vi "dfd_Validate Filter Bank.vi"(8 "error in (no error)":errorcluster, 11 "filter banks in":T1 {"mFBank_SynthesisFilters"."mMRate_SumWl" min=1 max=32 step=1; "mFBank_SynthesisFilters"."mMRate_InputIwl" min=1 max=32 step=1; "mFBank_SynthesisFilters"."mMRate_GainWl" min=1 max=32 step=1; "mFBank_SynthesisFilters"."mMRate_OutputWl" min=1 max=32 step=1; "mFBank_SynthesisFilters"."mMRate_InputWl" min=1 max=32 step=1; "mFBank_SynthesisFilters"."mMRate_CoefWl" min=1 max=32 step=1; "mFBank_SynthesisFilters"."mMRate_Mode" items=["Default"=-1, "No Rate Change"=0, "Interpolation"=1, "Decimation"=2, "Interpolated"=3, "Rational"=4]; "mFBank_AnalysisFilters"."mMRate_SumWl" min=1 max=32 step=1; "mFBank_AnalysisFilters"."mMRate_InputIwl" min=1 max=32 step=1; "mFBank_AnalysisFilters"."mMRate_GainWl" min=1 max=32 step=1; "mFBank_AnalysisFilters"."mMRate_OutputWl" min=1 max=32 step=1; "mFBank_AnalysisFilters"."mMRate_InputWl" min=1 max=32 step=1; "mFBank_AnalysisFilters"."mMRate_CoefWl" min=1 max=32 step=1; "mFBank_AnalysisFilters"."mMRate_Mode" items=["Default"=-1, "No Rate Change"=0, "Interpolation"=1, "Decimation"=2, "Interpolated"=3, "Rational"=4]; "mFBank_Type" items=["Uniform", "Non-Uniform"]}) -> (0 "error out":errorcluster, 2 "is Valid?":bool, 3 "filter bank out":T1 {"mFBank_SynthesisFilters"."mMRate_SumWl" min=1 max=32 step=1; "mFBank_SynthesisFilters"."mMRate_InputIwl" min=1 max=32 step=1; "mFBank_SynthesisFilters"."mMRate_GainWl" min=1 max=32 step=1; "mFBank_SynthesisFilters"."mMRate_OutputWl" min=1 max=32 step=1; "mFBank_SynthesisFilters"."mMRate_InputWl" min=1 max=32 step=1; "mFBank_SynthesisFilters"."mMRate_CoefWl" min=1 max=32 step=1; "mFBank_SynthesisFilters"."mMRate_Mode" items=["Default"=-1, "No Rate Change"=0, "Interpolation"=1, "Decimation"=2, "Interpolated"=3, "Rational"=4]; "mFBank_AnalysisFilters"."mMRate_SumWl" min=1 max=32 step=1; "mFBank_AnalysisFilters"."mMRate_InputIwl" min=1 max=32 step=1; "mFBank_AnalysisFilters"."mMRate_GainWl" min=1 max=32 step=1; "mFBank_AnalysisFilters"."mMRate_OutputWl" min=1 max=32 step=1; "mFBank_AnalysisFilters"."mMRate_InputWl" min=1 max=32 step=1; "mFBank_AnalysisFilters"."mMRate_CoefWl" min=1 max=32 step=1; "mFBank_AnalysisFilters"."mMRate_Mode" items=["Default"=-1, "No Rate Change"=0, "Interpolation"=1, "Decimation"=2, "Interpolated"=3, "Rational"=4]; "mFBank_Type" items=["Uniform", "Non-Uniform"]})   [LabVIEW 2017, in "NI_DigFilter_FilterBank.lvlib"]
uses:
  <vilib>/addons/Digital Filter Design/NI_DigFilter_FilterBank.lvlib
  <vilib>/addons/Digital Filter Design/FilterBank.llb/Object/DFD Filter Bank Obj.ctl
  <vilib>/addons/Digital Filter Design/_Objects.llb/DFD Multirate Filter Obj.ctl
  <vilib>/addons/Digital Filter Design/_Objects.llb/DFD Multirate Mode.ctl
  <vilib>/addons/Digital Filter Design/_Objects.llb/DFD Coef Norm Type.ctl
  <vilib>/addons/Digital Filter Design/_Objects.llb/DFD Round-off Mode.ctl
  <vilib>/addons/Digital Filter Design/_Objects.llb/DFD FXP MRate Multiply Mode.ctl
  <vilib>/addons/Digital Filter Design/FilterBank.llb/Object/DFD Filter Bank Processing Method.ctl
  <vilib>/addons/Digital Filter Design/FilterBank.llb/Object/DFD Filter Bank Type.ctl
  <vilib>/addons/Digital Filter Design/_Misc.llb/dfd_Error Handlers (Single).vi
  <vilib>/addons/Digital Filter Design/NI_DigFilterLicensed.lvlib
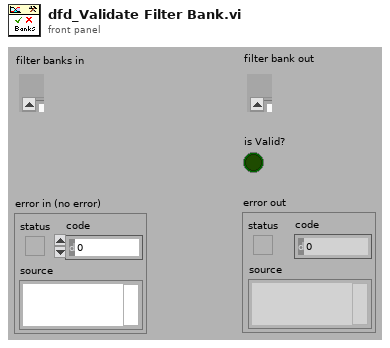
[diagram p1: front panel]
types:
  T1 = typedef "NI_DigFilter_FilterBank.lvlib/DFD Filter Bank Obj.ctl" = cluster{"mFBank_AnalysisFilters":T2[], "mFBank_SynthesisFilters":T2[], "mFBank_#Bands":i32, "mFBank_ProcMethod":T7, "mFBank_Coeffs":dbl[], "mFBank_Gain":dbl, "mFBank_Delay":i32, "mFBank_Type":T8}
  T2 = typedef "NI_DigFilterLicensed.lvlib/DFD Multirate Filter Obj.ctl" = cluster{"mMRate_Structure":enum16{"CIC", "FIR", "IIR", "Lattice"}, "mMRate_Mode":T3, "mMRate_Factor":i32, "mMRate_FIRParams":cluster{"mMRate_FIR_H":dbl[], "mMRate_FIR_IsNyquist?":bool, "mMRate_FIR_IsSymmetric?":bool}, "mMRate_CICParams":cluster{"mMRate_CIC_#Stage":i32, "mMRate_CIC_Lag":i32, "mMRate_CIC_Type":enum16{"Lowpass", "Highpass"}}, "mMRate_Order":i32, "mMRate_Version":string, "mMRate_Comments":string, "mMRate_RationalFactor":cluster{"mMRate_L":i32, "mMRate_M":i32}, "mMRate_Fs":dbl, "mMRate_Quantized?":bool, "mMRate_QFilterGain":dbl, "mMRate_CoefWl":i16, "mMRate_Scaling":cluster{"mMRate_ScaleByPowerOf2?":bool, "mMRate_ScaleType":T4}, "mMRate_InputWl":i16, "mMRate_OutputWl":i16, "mMRate_OutputMode":T5, "mMRate_MultMode":T6, "mMRate_BitPruning":bool, "mMRate_GainWl":i16, "mMRate_OutputFwl":i16, "mMRate_SumIwl":i16, "mMRate_InputIwl ":i16, "mMRate_SumWl":i16, "mMRate_CoefIwl":i16}
  T3 = typedef "NI_DigFilterLicensed.lvlib/DFD Multirate Mode.ctl" = i16
  T4 = typedef "NI_DigFilterLicensed.lvlib/DFD Coef Norm Type.ctl" = enum16{"No Norm", "Time Domain 1-Norm", "Time Domain 2-Norm", "Time Domain Inf-Norm"}
  T5 = typedef "NI_DigFilterLicensed.lvlib/DFD Round-off Mode.ctl" = enum16{"Nearest", "Truncation"}
  T6 = typedef "NI_DigFilterLicensed.lvlib/DFD FXP MRate Multiply Mode.ctl" = enum16{"Truncated", "Full"}
  T7 = typedef "NI_DigFilter_FilterBank.lvlib/DFD Filter Bank Processing Method.ctl" = enum16{"General", "2-Band QMF Lattice", "Cosine-Modulated"}
  T8 = typedef "NI_DigFilter_FilterBank.lvlib/DFD Filter Bank Type.ctl" = u16
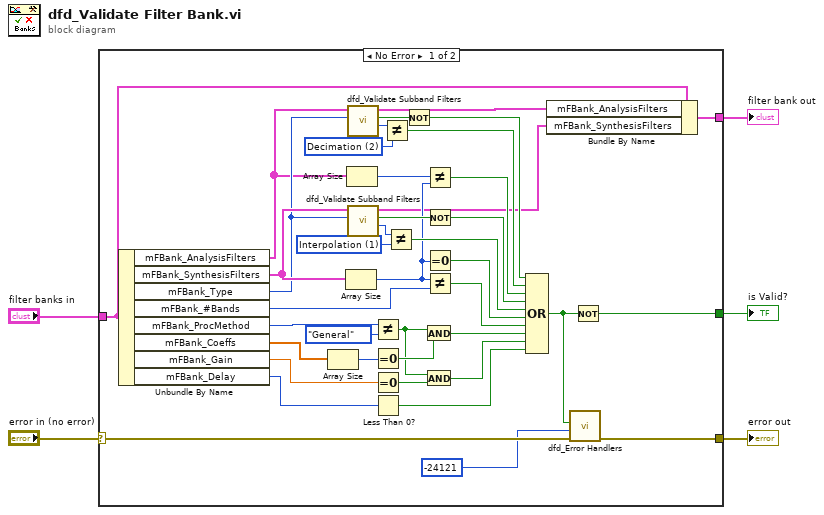
[diagram p0: block diagram]
diagram:
  n1 = case shown="No Error" "error in (no error)" {
    selector: "error in (no error)" -> [w36 w47]
    tunnel: "filter banks in" -> [w10 w46]
    tunnel: [w37 w47] -> w3
    tunnel: [w33 _] -> w2
    tunnel: [w6 w46] -> w1
    frame No Error {
      w25 = T3 1 items=["Default"=-1, "No Rate Change"=0, "Interpolation"=1, "Decimation"=2, "Interpolated"=3, "Rational"=4] ("y")
      w29 = T3 2 items=["Default"=-1, "No Rate Change"=0, "Interpolation"=1, "Decimation"=2, "Interpolated"=3, "Rational"=4] ("y")
      n2 = Unbundle By Name(w10) -> ("mFBank_AnalysisFilters"=w8:T2[], "mFBank_SynthesisFilters"=w32:T2[], "mFBank_Type"=w27:T8, "mFBank_#Bands"=w45:i32, "mFBank_ProcMethod"=w44:T7, "mFBank_Coeffs"=w43:dbl[], "mFBank_Gain"=w42:dbl, "mFBank_Delay"=w41:i32)
      n3 = Array Size(array=w43) -> (size(s)=w19:i32)
      n4 = Array Size(array=w32) -> (size(s)=w12:i32)
      n5 = Array Size(array=w8) -> (size(s)=w13:i32)
      n6 = call <vilib>:"dfd_Validate Subband Filters.vi"("filter bank structure"=w27, "subband filters in"=w8) -> ("filter mode"=w30:T3, "is Valid?"=w28:bool, "subband filters out"=w9:T2[])  [unwired: 6 in, 1 out]
      n7 = call <vilib>:"dfd_Validate Subband Filters.vi"("filter bank structure"=w27, "subband filters in"=w32) -> ("filter mode"=w26:T3, "is Valid?"=w31:bool, "subband filters out"=w7:T2[])  [unwired: 6 in, 1 out]
      n8 = Not Equal?(x=w44, y=DFD_Filter_Bank_Processing_Method."General") -> (x != y?=w16:bool)
      n9 = Equal To 0?(x=w19) -> (x = 0?=w18:bool)
      n10 = Equal To 0?(x=w42) -> (x = 0?=w17:bool)
      n11 = Less Than 0?(x=w41) -> (x < 0?=w15:bool)
      n12 = Not Equal?(x=w30, y=w29) -> (x != y?=w23:bool)
      n13 = Not Equal?(x=w26, y=w25) -> (x != y?=w21:bool)
      n14 = Not(x=w28) -> (.not. x?=w24:bool)
      n15 = And(x=w16, y=w18) -> (x .and. y?=w40:bool)
      n16 = And(x=w16, y=w17) -> (x .and. y?=w14:bool)
      n17 = Not Equal?(x=w13, y=w12) -> (x != y?=w11:bool)
      n18 = Not(x=w31) -> (.not. x?=w22:bool)
      n19 = Equal To 0?(x=w12) -> (x = 0?=w38:bool)
      n20 = Not Equal?(x=w12, y=w45) -> (x != y?=w39:bool)
      n21 = Compound Arithmetic op=OR(w24, w23, w11, w22, w21, w38, w39, w40, w14, w15) -> (w34:bool)
      n22 = Bundle By Name(cluster=w10, "mFBank_AnalysisFilters"=w9, "mFBank_SynthesisFilters"=w7) -> (w6:T1)
      n23 = call-poly <vilib>:"dfd_Error Handlers.vi"("error in (no error)"=w36, "error code"=-24121 ("ERR_INVALID_FILTERBANK_OBJ"), "condition failed?"=w34) -> ("error out"=w37:errorcluster)  [unwired: 8 in]
      n24 = Not(x=w34) -> (.not. x?=w33:bool)
    }
    frame Error {
    }
  }
  "filter bank out" <- w1
  "error out" <- w3
  "is Valid?" <- w2
